vi "SetAzCamParameter.vi"(1 "Value":string, 2 "Parameter":string) -> (0 "Error":bool)   [LabVIEW 2014]
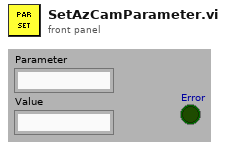
[diagram p1: front panel]
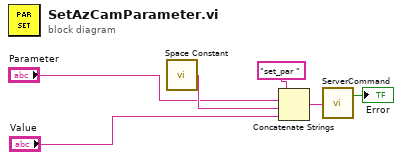
[diagram p0: block diagram]
diagram:
  n1 = call <vilib>:"Space Constant.vi"() -> ("String"=w3:string)
  n2 = Concatenate Strings("set_par " ("Attribute"), "Parameter", w3, "Value") -> (w6:string)
  n3 = call "ServerCommand.vi"("Command"=w6) -> ("Error"=→"Error":bool)  [unwired: 1 out]
